vi "LJT4_stream_start.vi"(7 "Scan List":string[](array[string]), 8 "error in":errorcluster, 9 "Read Rate (Hz)":dbl, 10 "Scan Rate (Hz)":dbl, 11 "Handle in":i32) -> (0 "error out":errorcluster, 1 "NumReadAddresses":i32, 2 "ScansPerRead Out":i32, 3 "Handle out":i32, 4 "Actual SampleRate":dbl, 5 "ScansPerRead":i32)   [LabVIEW 2019]
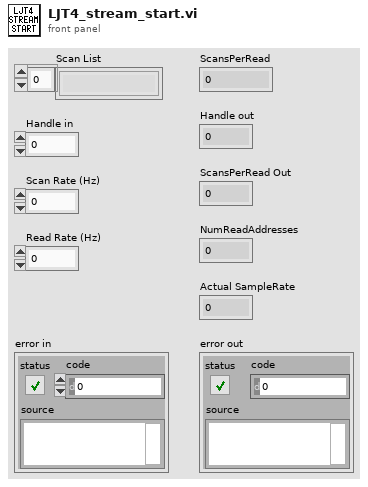
[diagram p1: front panel]
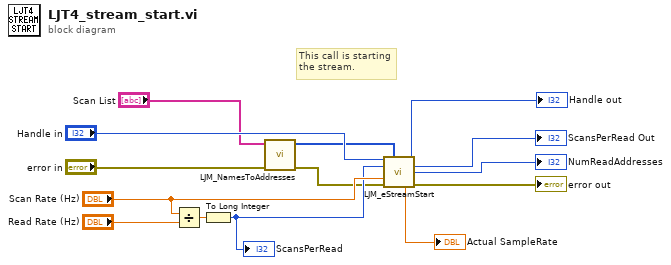
[diagram p0: block diagram]
diagram:
  # "This call is starting\nthe stream."
  n1 = Divide(x="Scan Rate (Hz)", y="Read Rate (Hz)") -> (x/y=w5:dbl)
  n2 = To Long Integer(number=w5) -> (32bit integer=w6:i32)
  "ScansPerRead" <- w6
  n3 = call "LJM_NamesToAddresses.vi"("error in"="error in", "aNames"="Scan List") -> ("error out"=w3:errorcluster, "aAddresses"=w8:i32[])  [unwired: 7 in, 1 out]
  n4 = call "LJM_eStreamStart.vi"("Handle In"="Handle in", "aScanList"=w8, "ScansPerRead"=w6, "ScanRate"="Scan Rate (Hz)", "error in"=w3) -> ("Handle Out"=→"Handle out":i32, "ScansPerRead Out"=→"ScansPerRead Out":i32, "NumReadAddresses"=→"NumReadAddresses":i32, "Actual SampleRate"=→"Actual SampleRate":dbl, "error out"=→"error out":errorcluster)  [unwired: 5 in, 1 out]
